vi "check_ups.vi"() -> (0 "Error: no voltages read":bool, 1 "Timestamp last measured":timestamp, 2 "Last date-time measured":string, 3 "Minimum input voltage measured":dbl)   [LabVIEW 2012]
uses:
  <vilib>/Utility/file.llb/Read From Spreadsheet File (string).vi
panel:
  out "Array 2":string[](array[string])
  out "Array":dbl[](array[numeric])
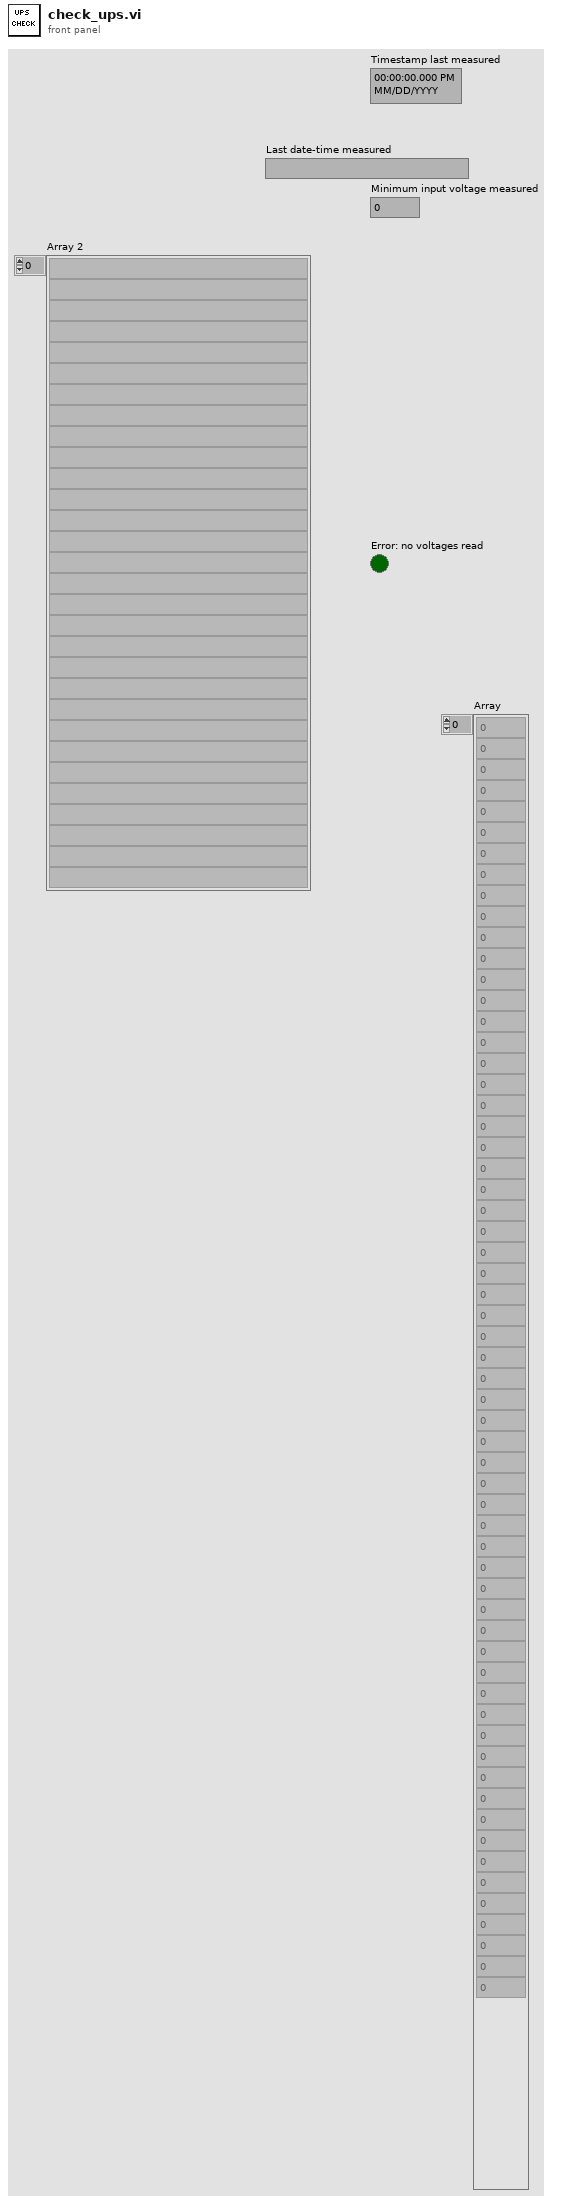
[diagram p1: front panel]
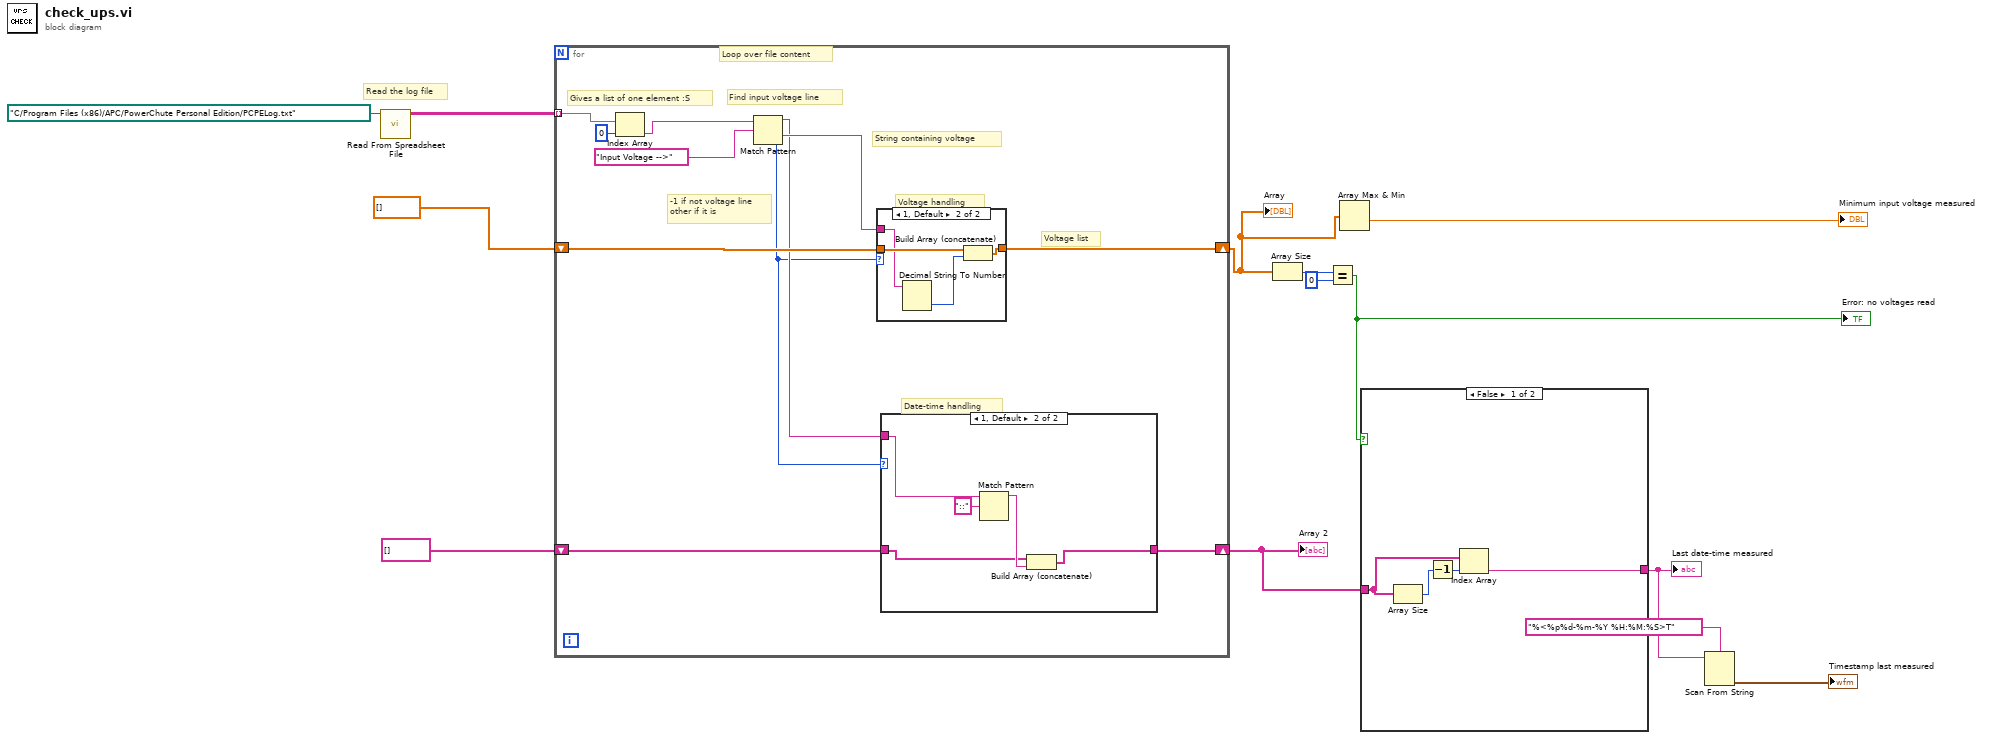
[diagram p0: block diagram]
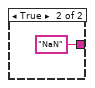
[diagram p2: hidden frame]
diagram:
  # "Read the log file"
  n1 = call-poly <vilib>:"Read From Spreadsheet File.vi"("file path (dialog if empty)"=path "C:/Program Files (x86)/APC/PowerChute Personal Edition/PCPELog.txt") -> ("all rows"=w12:string[][])  [unwired: 6 in, 4 out]
  n2 = for {
    tunnel: w12 -> [w24] mode=indexing
    shift-right: [w18] -> w7
    shift-left: dbl[] [] -> [w20]
    shift-right: [w15] -> w5
    shift-left: string[] [] -> [w14]
    # "Date-time handling"
    # "Voltage handling"
    # "Voltage list"
    # "-1 if not voltage line\nother if it is"
    # "String containing voltage"
    # "Find input voltage line"
    # "Loop over file content"
    # "Gives a list of one element :S"
    n3 = Index Array(array=w24, index=0) -> (element=w22:string)
    n4 = Match Pattern(string=w22, regular expression="Input Voltage -->") -> (before substring=w17:string, after substring=w19:string, offset past match=w16:i32)  [unwired: 1 in, 1 out]
    n5 = case shown="1, Default" w16 {
      tunnel: w20 -> [w31 w35]
      tunnel: w19 -> [_ w34]
      tunnel: [w31 w32] -> w18
      frame -1 {
      }
      frame 1, Default {
        n6 = Decimal String To Number(string=w34) -> (number=w33:i32)  [unwired: 2 in, 1 out]
        n7 = Build Array (concatenate)(w35, w33) -> (w32:dbl[])
      }
    }
    n8 = case shown="1, Default" w16 {
      tunnel: w17 -> [_ w30]
      tunnel: [w25 w26] -> w15
      tunnel: w14 -> [w25 w27]
      frame -1 {
      }
      frame 1, Default {
        n9 = Match Pattern(string=w30, regular expression="::") -> (before substring=w28:string)  [unwired: 1 in, 3 out]
        n10 = Build Array (concatenate)(w27, w28) -> (w26:string[])
      }
    }
  }
  "Array" <- w7
  "Array 2" <- w5
  n11 = Array Size(array=w7) -> (size(s)=w10:i32)
  n12 = Equal?(x=w10, y=0) -> (x = y?=w6:bool)
  "Error: no voltages read" <- w6
  n13 = Array Max & Min(array=w7) -> (min value=→"Minimum input voltage measured":dbl)  [unwired: 3 out]
  n14 = case shown="False" w6 {
    tunnel: w5 -> [w39 _]
    tunnel: [w37 "NaN"] -> w3
    frame False {
      n15 = Array Size(array=w39) -> (size(s)=w38:i32)
      n16 = Decrement(x=w38) -> (x-1=w36:i32)
      n17 = Index Array(array=w39, index=w36) -> (element=w37:string)
    }
    frame True {
    }
  }
  "Last date-time measured" <- w3
  n18 = Scan From String(format string="%<%p%d-%m-%Y %H:%M:%S>T", input string=w3) -> (output 1=→"Timestamp last measured":timestamp)  [unwired: 3 in, 3 out]
